vi "myRIO_BRig DIO Block Read.vi"(6 "ENA":bool, 7 "Divisor":u16, 8 "DIR":bool, 9 "OUT":bool, 10 "FIFO In":refnum<k21>="DI DMA", 11 "DIO Refnum":refnum<k21>) -> (1 "Timed Out?":bool, 3 "IN":bool)   [LabVIEW 2014]
uses:
  <vilib>/rvi/eio/common/nirviEmuReportErrorAndStop.vi
  <vilib>/rvi/interface/RandomDataEmulation/niFpgaRandomDataHandleErrors.vi
  <vilib>/rvi/Emulation/niFpgaProcessEmulError.vi
  <vilib>/rvi/FIFO/Fifo_Resource/nirvififoEmulationSetSize.vi
  <vilib>/rvi/DataTransferAndStorage/Container/Common/niFpgaContainerGetUniqueNameForEmu.vi
  <vilib>/rvi/FIFO/Fifo_Resource/nirviFifoEmulationQueueMgr.vi
  <instcachedir>/0/nirviFifoEmulationQueueMgr_E5CAEC123FF24DC58D834DCA3CDAA9B5.lvgen/nirviFifoEmulationQueueMgr_E5CAEC123FF24DC58D834DCA3CDAA9B5_001.vi
  <vilib>/rvi/Emulation/niFpgaEmulationIsFPGAContextNoSignature.vi
  <vilib>/rvi/errors/nirviReportUnexpectedCaseInternalError.vi
  <vilib>/rvi/errors/nirviReportUnexpectedCaseInternalError (U32).vi
  <vilib>/rvi/occurrence/nirviWaitOnOccurrenceBase.vi
  <vilib>/rvi/FIFO/Fifo_Resource/nirvififoEmulationReleaseLock.vi
  <vilib>/rvi/FIFO/Fifo_Resource/nirvififoEmulationObtainLock.vi
  <vilib>/rvi/FIFO/Fifo_Resource/nirvififoEmulationCreateLock.vi
  <vilib>/rvi/errors/niFpgaSetErrorForExecOnDevCompSimple.vi
  <vilib>/rvi/Emulation/niFpgaSctlEmulationGetInTimedLoop.vi
  <vilib>/rvi/FIFO/Fifo_Resource/nirvififoEmulationDetermineInputValidOut.vi
  <vilib>/rvi/DataTransferAndStorage/Container/Common/niFpgaContainerExecOnDevCompGetState.vi
  <vilib>/rvi/DataTransferAndStorage/Container/XNode/niFpgaContainer.xnode
  <vilib>/rvi/FIFO/Fifo_Resource/niFpgaFifoEmulationRefIn.vi
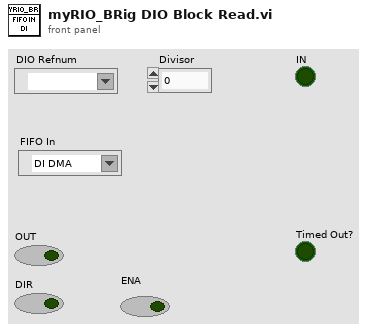
[diagram p1: front panel]
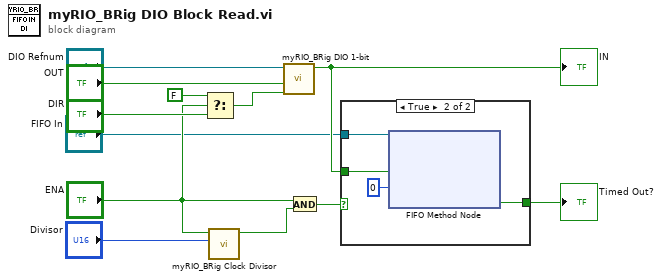
[diagram p0: block diagram]
diagram:
  n1 = Select(t=FALSE ("Flag"), s="ENA", f="DIR") -> (s? t:f=w6:bool)
  n2 = call "myRIO_BRig Clock Divisor.vi"("Count Number"="Divisor", "Trigger"="ENA") -> ("Finished"=w2:bool)  [unwired: 9 in]
  n3 = call "myRIO_BRig DIO 1-bit.vi"("DIR"=w6, "OUT"="OUT", "DIO Refnum"="DIO Refnum") -> ("IN"=w9:bool)  [unwired: 8 in]
  "IN" <- w9
  n4 = And(x="ENA", y=w2) -> (x .and. y?=w5:bool)
  n5 = case shown="True" w5 {
    tunnel: w9 -> [_ w16]
    tunnel: [_ w14] -> w12
    tunnel: "FIFO In" -> [_ w13]
    frame False {
    }
    frame True {
      n6 = xnode ("FIFO Method Node")("Element"=w16, "Timeout"=0, "FIFO In"=w13) -> ("Timed Out?"=w14:bool)  [unwired: 1 out]
    }
  }
  "Timed Out?" <- w12
